vi "armpotauto.vi"() -> ()   [LabVIEW 2015]
panel:
  out "Pot For arm":dbl
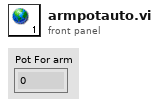
[diagram p1: front panel]
diagram:
